vi "Trial Start flag initialise.vi"(8 "error in (no error)":errorcluster) -> (0 "error out (no error)":errorcluster)   [LabVIEW 2020]
uses:
  typedefs/Functions enum.ctl
  <vilib>/Utility/error.llb/DialogType.ctl
  Global Variables/General Globals.vi
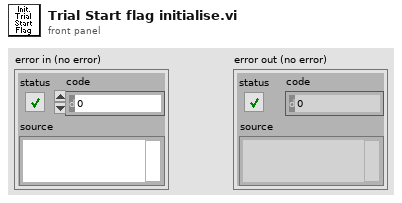
[diagram p1: front panel]
types:
  T1 = typedef "Functions enum.ctl" = enum16{"Create", "Start", "Write", "Stop", "Clear"}
  T2 = typedef "DialogType.ctl" = u16
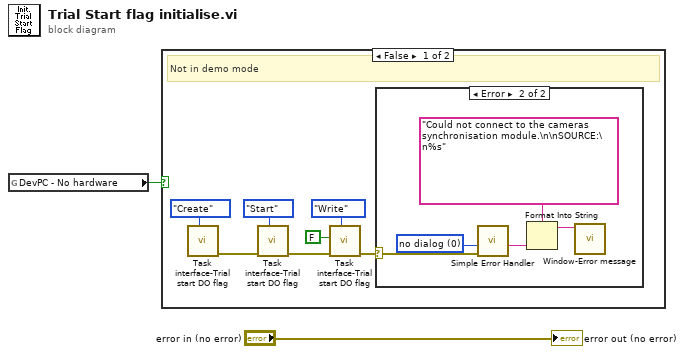
[diagram p0: block diagram]
diagram:
  n1 = global read "General Globals.vi" "DevPC - No hardware"() -> (w1:bool)
  n2 = case shown="False" w1 {
    frame False {
      # "Not in demo mode"
      n3 = call "Task interface-Trial start DO flag.vi"("Function"=Functions_enum."Create") -> ("error out"=w6:errorcluster)  [unwired: 10 in]
      n4 = call "Task interface-Trial start DO flag.vi"("Function"=Functions_enum."Start", "error in"=w6) -> ("error out"=w8:errorcluster)  [unwired: 9 in]
      n5 = call "Task interface-Trial start DO flag.vi"("Function"=Functions_enum."Write", "error in"=w8, "DO value"=FALSE) -> ("error out"=w3:errorcluster)  [unwired: 8 in]
      n6 = case shown="Error" w3 {
        selector: w3 -> [_ w14]
        frame No Error {
        }
        frame Error {
          w13 = T2 0 items=["no dialog", "OK message", "continue or stop message", "OK message + warnings", "continue/stop + warnings"] ("type of dialog (OK msg:1)")
          n7 = call <vilib>:"Simple Error Handler.vi"("type of dialog (OK msg:1)"=w13, "error in (no error)"=w14) -> ("source out"=w12:string)  [unwired: 3 in, 4 out]
          n8 = Format Into String(format string="Could not connect to the cameras synchronisation module.\n\nSOURCE:\n%s" ("Error Source"), w12) -> (resulting string=w10:string)  [unwired: 2 in, 1 out]
          n9 = call "Window-Error message.vi"("Message"=w10) -> ()  [unwired: 10 in, 1 out]
        }
      }
    }
    frame True {
      # "Demo mode"
    }
  }
  "error out (no error)" <- "error in (no error)"
